vi "Define.vi"(11 "Definition":T1) -> (3 "DateTime out":refnum<class "Timestamp.lvclass">)   [LabVIEW 2020, in "Conditum.lvlib" / "Columns.lvlib" / "Timestamp.lvclass"]
uses:
  Timestamp.lvclass
  C:/dev/lv20CE/lv-conditum/Conditum/Columns/Type/Type.lvclass
  Timestamp Definition.ctl
  Type/Definition.ctl
  Attributes.ctl
  Definition.ctl
  Field Type.ctl
  Type/Type.lvclass/Type.ctl
  Timestamp.lvclass/Timestamp.ctl
  Type/Type.lvclass
  Conditum.lvlib
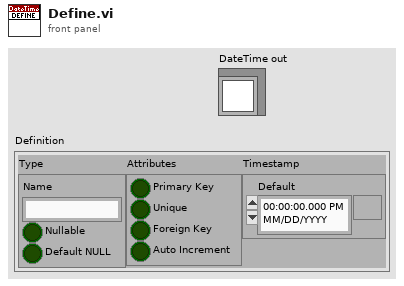
[diagram p1: front panel]
types:
  T1 = typedef "Conditum.lvlib/Columns.lvlib/Timestamp.lvclass/Timestamp Definition.ctl" = cluster{"Type":T2, "Attributes":T3, "Timestamp":T4}
  T2 = typedef "Conditum.lvlib/Columns.lvlib/Type.lvclass/Definition.ctl" = cluster{"Name":string, "Nullable":bool, "Default NULL":bool}
  T3 = typedef "Conditum.lvlib/Attributes.ctl" = cluster{"Primary Key":bool, "Unique":bool, "Foreign Key":bool, "Auto Increment":bool}
  T4 = typedef "Conditum.lvlib/Columns.lvlib/Timestamp.lvclass/Definition.ctl" = cluster{"Default":timestamp}
  T5 = typedef "Conditum.lvlib/Field Type.ctl" = enum16{"None", "ID", "Boolean", "Integer", "Double", "Timestamp", "String", "Text", "Entity"}
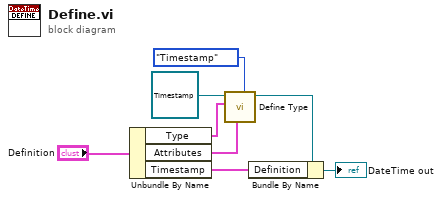
[diagram p0: block diagram]
diagram:
  n1 = Unbundle By Name("Definition") -> ("Type"=w6:T2, "Attributes"=w2:T3, "Timestamp"=w5:T4)
  n2 = call "Define Type.vi"("Type"=Field_Type."Timestamp", "Attributes"=w2, "Definition"=w6, "Type in"=refnum<class "Timestamp.lvclass"> refnum ("DateTime out")) -> ("Type out"=w4:refnum<class "Timestamp.lvclass">)  [unwired: 7 in]
  n3 = Bundle By Name(cluster=w4, "Definition"=w5) -> (→"DateTime out":refnum<class "Timestamp.lvclass">)
